vi "PCO_SetBinning.vi"(8 "error in (no error)":errorcluster {"code" format="%x"}, 9 "wBinVert":u16, 10 "wBinHorz":u16, 11 "ph":u64) -> (0 "error out":errorcluster {"code" format="%x"}, 2 "ErrorMessage":i32 format="%x", 3 "ph out":u64)   [LabVIEW 2019, in "SDK.lvlib" / "ImageSensor.lvlib"]
doc: "<b>Description:</b>\nThis function does set the horizontal and vertical binning of the camera. Possible values can be calculated from the binning parameter in the PCO_Description structure. If the binning settings are changed, the ROI (region of interest) setting must be adapted, before PCO_ArmCamera is called. See chapter IMAGE AREA SELECTION (ROI).\nInvalid values result in a failure response message.\nThe command will be rejected, if Recording State is [run], see PCO_GetRecordingState.\n\n<b>Supported camera type:</b>\nAll cameras\n\n<b>Descriptor dependency:</b>\nNone"
uses:
  ImageSensor.lvlib
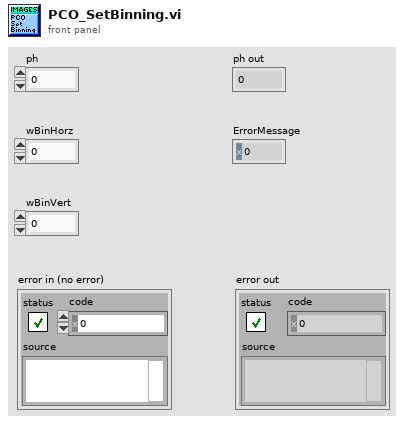
[diagram p1: front panel]
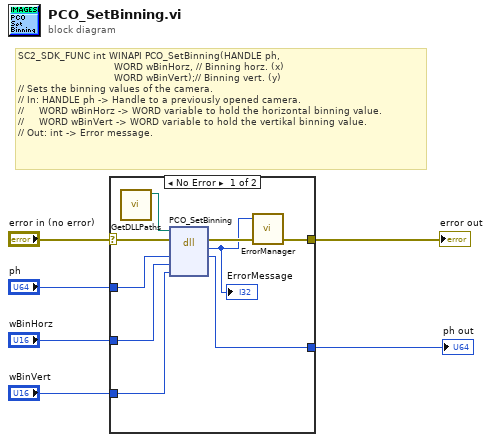
[diagram p0: block diagram]
diagram:
  # "SC2_SDK_FUNC int WINAPI PCO_SetBinning(HANDLE ph,\n                                WORD wBinHorz, // Binning horz. (x)\n                                WORD wBinVert);// Binning vert. (y)\n// Sets the binning values of the camera.\n// In: HANDLE ph -> Handle to a previously opened camera.\n//     WORD wBinHorz -> WORD variable to hold the horizontal binning value.\n//     WORD wBinVert -> WORD variable to hold the vertikal binning value.\n// Out: int -> Error message."
  n1 = case shown="No Error" "error in (no error)" {
    selector: "error in (no error)" -> [w11 w17]
    tunnel: "ph" -> [w15 w16]
    tunnel: [w14 w16] -> w5
    tunnel: "wBinHorz" -> [w13 _]
    tunnel: "wBinVert" -> [w12 _]
    tunnel: [w9 w17] -> w2
    frame No Error {
      n2 = call "GetDLLPaths.vi"() -> ("SC2_Cam_Path"=w7:path)  [unwired: 8 in, 3 out]
      n3 = dll-call lib="?" fn="PCO_SetBinning"(path in=w7, error in=w11, "ph"=w15, "wBinHorz"=w13, "wBinVert"=w12) -> (error out=w10:errorcluster, "return type"=w8:i32, "ph"=w14:u64)  [unwired: 3 in, 1 out]
      "ErrorMessage" <- w8
      n4 = call "ErrorManager.vi"("error in (no error)"=w10, "error code"=w8) -> ("error out"=w9:errorcluster)  [unwired: 2 in, 1 out]
    }
    frame Error {
    }
  }
  "ph out" <- w5
  "error out" <- w2
